vi "_Parse Instrument Channel_libESP301.vi"(11 "Instrument Channel":string="GPIB/0:4,0") -> (0 "T - GPIB, F - RS232":bool, 1 "Hardware Address":i32, 2 "Instrument Address":i16, 3 "Instrument Channel out":string="GPIB/0:4,0", 5 "Valid String":bool)   [LabVIEW 2019, in "Newport ESP301.lvlib"]
doc: "Instrument Channel string is parsed into its components.\n\nIf channel string is a plain integer, it is sent on as a GPIB channel."
uses:
  Newport ESP301.lvlib
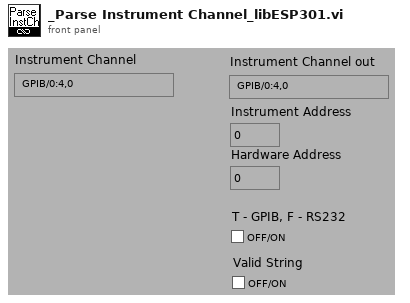
[diagram p1: front panel]
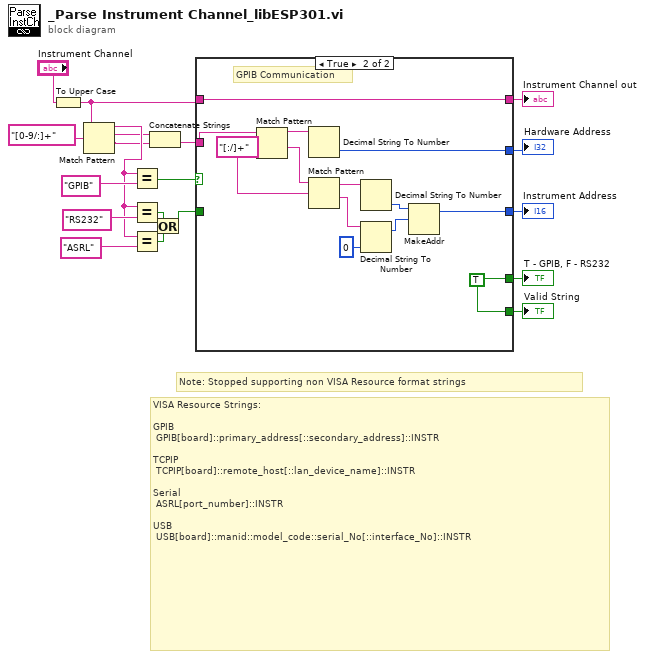
[diagram p0: block diagram]
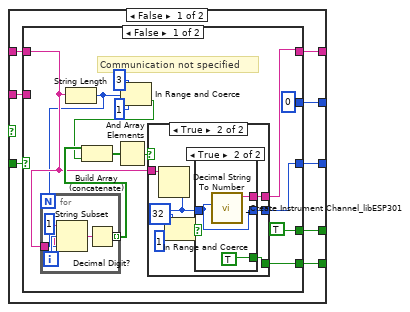
[diagram p2: hidden frame]
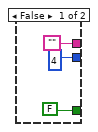
[diagram p3: hidden frame]
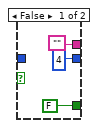
[diagram p4: hidden frame]
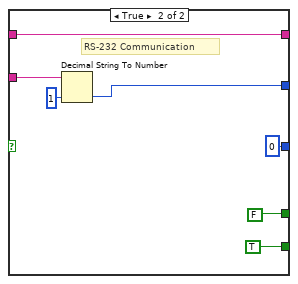
[diagram p5: hidden frame]
diagram:
  # "Note: Stopped supporting non VISA Resource format strings"
  # "VISA Resource Strings:\n\nGPIB\n GPIB[board]::primary_address[::secondary_address]::INSTR\n \nTCPIP\n TCPIP[board]::remote_host[::lan_device_name]::INSTR\n \nSerial\n ASRL[port_number]::INSTR\n \nUSB\n USB[board]::manid::model_code::serial_No[::interface_No]::INSTR"
  n1 = To Upper Case(1:"Instrument Channel") -> (0:w2:string)
  n2 = Match Pattern(string=w2, regular expression="[0-9/:]+") -> (before substring=w5:string, match substring=w4:string, after substring=w3:string)  [unwired: 1 in, 1 out]
  n3 = Equal?(x=w5, y="GPIB") -> (x = y?=w17:bool)
  n4 = Equal?(x=w5, y="RS232") -> (x = y?=w9:bool)
  n5 = Equal?(x=w5, y="ASRL") -> (x = y?=w8:bool)
  n6 = Concatenate Strings(w4, w3) -> (w6:string)
  n7 = Or(x=w9, y=w8) -> (x .or. y?=w7:bool)
  n8 = case shown="True" w17 {
    tunnel: w6 -> [w26 w82]
    tunnel: w7 -> [w27 _]
    tunnel: [w25 w74] -> w15
    tunnel: [w20 w73] -> w16
    tunnel: [w24 w72] -> w14
    tunnel: [w23 w72] -> w13
    tunnel: w2 -> [w22 w71]
    tunnel: [w21 w71] -> w12
    frame False {
      n9 = case shown="False" w27 {
        tunnel: w26 -> [_ w69]
        tunnel: [0 w67] -> w25
        tunnel: [w28 TRUE] -> w24
        tunnel: [TRUE FALSE] -> w23
        tunnel: w22 -> [w30 w64]
        tunnel: [w34 w64] -> w21
        tunnel: [w33 0] -> w20
        frame False {
          # "Communication not specified"
          n10 = String Length(string=w30) -> (length=w29:i32)
          n11 = for {
            N: w29 -> [_]
            tunnel: [w42] -> w32 mode=indexing
            tunnel: w30 -> [w41]
            i -> [w44]
            n12 = String Subset(string=w41, offset (0)=w44, length (rest)=1) -> (substring=w45:string)
            n13 = Decimal Digit?(1:w45) -> (0:w42:bool)
          }
          n14 = In Range and Coerce(upper limit=3, x=w29, lower limit=1) -> (In Range?=w31:bool)  [unwired: 1 out]
          n15 = Build Array (concatenate)(w32, w31) -> (w36:bool[])
          n16 = And Array Elements(Boolean array=w36) -> (logical AND=w35:bool)
          n17 = case shown="True" w35 {
            tunnel: w30 -> [_ w56]
            tunnel: ["" w51] -> w34
            tunnel: [4 w50] -> w33
            tunnel: [FALSE w49] -> w28
            frame False {
            }
            frame True {
              n18 = Decimal String To Number(string=w56) -> (number=w53:i32)  [unwired: 2 in, 1 out]
              n19 = In Range and Coerce(upper limit=32, x=w53, lower limit=1) -> (In Range?=w52:bool)  [unwired: 1 out]
              n20 = case shown="True" w52 {
                tunnel: w53 -> [_ w61]
                tunnel: ["" w62] -> w51
                tunnel: [4 w61] -> w50
                tunnel: [FALSE TRUE] -> w49
                frame False {
                }
                frame True {
                  n21 = call "_Create Instrument Channel_libESP301.vi"("GPIB Primary Address (4)"=w61) -> ("Instrument Channel out"=w62:string)  [unwired: 8 in, 2 out]
                }
              }
            }
          }
        }
        frame True {
          # "RS-232 Communication"
          n22 = Decimal String To Number(string=w69, default (0L)=1) -> (number=w67:i32)  [unwired: 1 in, 1 out]
        }
      }
    }
    frame True {
      w72 = TRUE
      w70 = "[:/]+"
      # "GPIB Communication"
      n23 = Match Pattern(string=w82, regular expression=w70) -> (before substring=w81:string, after substring=w80:string)  [unwired: 1 in, 2 out]
      n24 = Decimal String To Number(string=w81) -> (number=w74:i32)  [unwired: 2 in, 1 out]
      n25 = Match Pattern(string=w80, regular expression=w70) -> (before substring=w79:string, after substring=w78:string)  [unwired: 1 in, 2 out]
      n26 = Decimal String To Number(string=w79) -> (number=w76:i32)  [unwired: 2 in, 1 out]
      n27 = Decimal String To Number(string=w78, default (0L)=0) -> (offset past number=w75:i32)  [unwired: 1 in, 1 out]
      n28 = MakeAddr(3:w75, 4:w76) -> (1:w73:i16)  [unwired: 1 in, 1 out]
    }
  }
  "Instrument Channel out" <- w12
  "Instrument Address" <- w16
  "Hardware Address" <- w15
  "T - GPIB, F - RS232" <- w13
  "Valid String" <- w14
